vi "Unwield.vi"(8 "Error In":errorcluster, 11 "reference in":refnum<class "Sword.lvclass">) -> (0 "Error Out":errorcluster, 3 "reference out":refnum<class "Sword.lvclass">)   [LabVIEW 2020, in "Sword.lvclass"]
uses:
  Sword.lvclass
  IEnchantment_interface/IEnchantment.lvclass
  Console_class/Console.lvclass
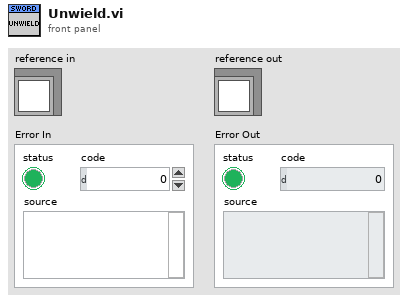
[diagram p1: front panel]
types:
  T1 = typedef "Sword.lvclass/ObjectAttributes.ctl" = cluster{"_enchantment":refnum<class "IEnchantment.lvclass">}
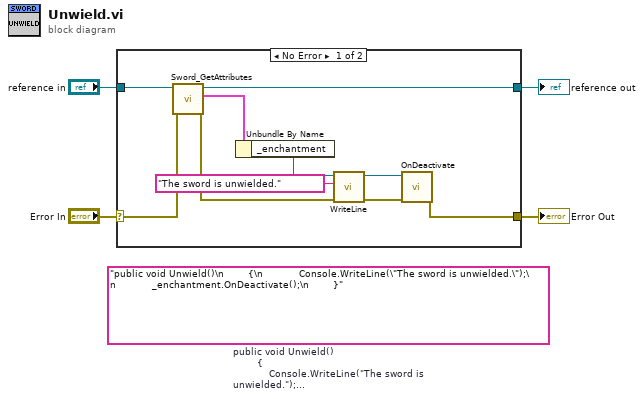
[diagram p0: block diagram]
diagram:
  (unwired) "public void Unwield()\n        {\n            Console.WriteLine(\"The sword is unwielded.\");\n            _enchantment.OnDeactivate();\n        }"  # public void Unwield()         {             Console.WriteLine("The sword is unwielded.");             _enchantment.OnDeactivate();         }
  n1 = case shown="No Error" "Error In" {
    selector: "Error In" -> [w6 w15]
    tunnel: [w5 w15] -> w3
    tunnel: [w7 w14] -> w1
    tunnel: "reference in" -> [w8 w14]
    frame No Error {
      n2 = call "Sword_GetAttributes.vi"("error in (no error)"=w6, "reference in"=w8) -> ("error out"=w11:errorcluster, "Data"=w13:T1, "reference out"=w7:refnum<class "Sword.lvclass">)  [unwired: 6 in, 1 out]
      n3 = Unbundle By Name(w13) -> ("_enchantment"=w12:refnum<class "IEnchantment.lvclass">)
      n4 = call "WriteLine.vi"("Error In"=w11, "ConsoleText"="The sword is unwielded.") -> ("Error Out"=w9:errorcluster)  [unwired: 9 in]
      n5 = call-dynamic "OnDeactivate.vi"("Error In"=w9, "object in"=w12) -> ("Error Out"=w5:errorcluster)  [unwired: 8 in, 1 out]
    }
    frame Error {
    }
  }
  "Error Out" <- w3
  "reference out" <- w1
